vi "Y Axis Speed Conversion.vi"() -> ()   [LabVIEW 2017]
panel:
  in  "Microsteps per Rev":T1(ring)
  out "Frequency (Hz)":dbl
  in  "Setpoint\nSpeed (mm/s)":dbl
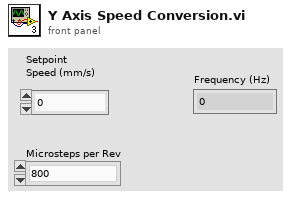
[diagram p1: front panel]
types:
  T1 = enum16{"800", "1600", "3200", "6400", "12800", "25600"}
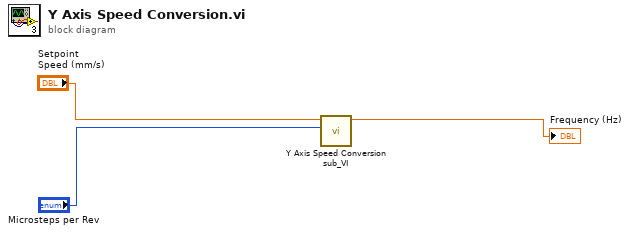
[diagram p0: block diagram]
diagram:
  n1 = call "Y Axis Speed Conversion sub_VI.vi"("Microsteps per Rev"="Microsteps per Rev", "Setpoint\nSpeed (mm/s)"="Setpoint\nSpeed (mm/s)") -> ("Numeric"=→"Frequency (Hz)":dbl)  [unwired: 9 in]
